vi "Log data.vi"(8 "error in (no error)":errorcluster, 11 "Vessel in":refnum<class "Vessel.lvclass">) -> (0 "error out":errorcluster, 3 "Vessel out":refnum<class "Vessel.lvclass">)   [LabVIEW 2014, in "Vessel.lvclass"]
uses:
  Vessel.lvclass
  <vilib>/imath/engines/lvmath/Plug In/_Char/NIMS_CH_character datatype.ctl
  <vilib>/imath/engines/lvmath2/RunTimeEngine/Managers/WorkSpace/UID Generator.vi
  <vilib>/imath/engines/lvmath/Plug In/_Char/NIMS_CH_String to Character Array.vi
  <vilib>/imath/engines/lvmath2/RunTimeEngine/BuiltInFunctions/length/NIMS_length(GV).vi
  <instcachedir>/0/NIMS_length(GV)_08A3D13377FD4E4B96F5795FBF3698FA.lvgen/NIMS_length(GV)_08A3D13377FD4E4B96F5795FBF3698FA_004.vi
  <vilib>/imath/engines/lvmath2/RunTimeEngine/RunTimeType/NIMS_RunTimeType_From StrictType (excl LVString).vi
  <instcachedir>/0/NIMS_RunTimeType_From StrictType (excl LVString)_15A5391EEA9C4AACB9955AC755B83D29.lvgen/NIMS_RunTimeType_From StrictType (excl LVString)_15A5391EEA9C4AACB9955AC755B83D29_000.vi
  <vilib>/imath/engines/lvmath2/RunTimeEngine/LocalVariableDefStatement/MC_LocalVariableDefStatement_Display.vi
  <vilib>/imath/engines/lvmath2/RunTimeEngine/RangeToken/NIMS_Range_R3 - Integer.vi
  <instcachedir>/0/NIMS_Range_R3 - Integer_66B9031982364693905FDE422E56E490.lvgen/NIMS_Range_R3 - Integer_66B9031982364693905FDE422E56E490_000.vi
  <vilib>/imath/engines/lvmath2/RunTimeEngine/CommandStatement/MC_CommandStatement_break.vi
  <vilib>/imath/engines/lvmath/Plug In/_Char/NIMS_CH_Character 2D to String 1D.vi
  <vilib>/imath/engines/lvmath2/RunTimeEngine/IndexRead/NIMS V(S).vi
  <instcachedir>/0/NIMS V(S)_0488751826AF41519A22953C041130DC.lvgen/NIMS V(S)_0488751826AF41519A22953C041130DC_003.vi
  <vilib>/imath/engines/lvmath2/RunTimeEngine/BuiltInFunctions/strcmp/NIMS_strcmp.vi
  <vilib>/imathl/engines/lvmath/Functions/Error Handling/Create Error.vi
  <vilib>/imath/engines/lvmath2/RunTimeEngine/VariableToken/NIMS_VariableToken_CondDefined.vi
  <instcachedir>/0/NIMS_VariableToken_CondDefined_EE8DD211A89249938CE6537267F5C9B3.lvgen/NIMS_VariableToken_CondDefined_EE8DD211A89249938CE6537267F5C9B3_003.vi
  <vilib>/imath/engines/lvmath2/RunTimeEngine/Managers/SymbolTable/Clear UID.vi
  <vilib>/imath/engines/lvmath2/RunTimeEngine/NodeEndStatement/NIMS_NodeEndStatement_Output.vi
  <instcachedir>/0/NIMS_NodeEndStatement_Output_53EC0D466D134D7ABD903AC30B43404B.lvgen/NIMS_NodeEndStatement_Output_53EC0D466D134D7ABD903AC30B43404B_011.vi
  <vilib>/imath/engines/lvmath2/RunTimeEngine/ErrorHandling/NIMS_Finalize Error.vi
  <vilib>/imath/engines/lvmath2/RunTimeEngine/IndexRead/NIMS V(R2).vi
  <instcachedir>/0/NIMS V(R2)_C76619605A0E4E9F8B2FA9389712AC47.lvgen/NIMS V(R2)_C76619605A0E4E9F8B2FA9389712AC47_002.vi
  <vilib>/imath/engines/lvmath/Plug In/_Char/NIMS_CH_Character RV to String.vi
  <instcachedir>/0/NIMS_NodeEndStatement_Output_53EC0D466D134D7ABD903AC30B43404B.lvgen/NIMS_NodeEndStatement_Output_53EC0D466D134D7ABD903AC30B43404B_009.vi
  Supervisor/Supervisor.lvclass
  <vilib>/imath/engines/lvmath2/RunTimeEngine/Managers/SymbolTable/NIMS_WorkSpace.lvlib
panel:
  out "log line OR":string="21:11:09.2343\t-0.00\t0.00\t30.00\t0.00\t0.00\t-0.00\t0.00\t0.01\t-0.01\t-0.00\t30.00\t0.00\t0.00\t-0.00\t0.00\t0.00\t0.00\t0.00\t30.00\t0.00\t0.00\t0.00\t0.00\t0.00\t132.54\t-43.98\t11.70\t-0.09\t-661 \t252 \t818 \t705 \r\n"
  out "appended path 2":path
  out "appended path":path
  out "log line camera":string="21:11:09.2343\t-0.00\t0.00\t30.00\t0.00\t0.00\t-0.00\t0.00\t0.01\t-0.01\t-0.00\t30.00\t0.00\t0.00\t-0.00\t0.00\t0.00\t0.00\t0.00\t30.00\t0.00\t0.00\t0.00\t0.00\t0.00\t132.54\t-43.98\t11.70\t-0.09\t-661 \t252 \t818 \t705 \r\n"
  out "Start New LogFile":bool
  out "path to log files":string
  out "path 2":path
  out "path":path
  out "log line tau":string="21:11:09.2343\t-0.00\t0.00\t30.00\t0.00\t0.00\t-0.00\t0.00\t0.01\t-0.01\t-0.00\t30.00\t0.00\t0.00\t-0.00\t0.00\t0.00\t0.00\t0.00\t30.00\t0.00\t0.00\t0.00\t0.00\t0.00\t132.54\t-43.98\t11.70\t-0.09\t-661 \t252 \t818 \t705 \r\n"
  out "log line nu":string="21:11:09.2343\t-0.00\t0.00\t30.00\t0.00\t0.00\t-0.00\t0.00\t0.01\t-0.01\t-0.00\t30.00\t0.00\t0.00\t-0.00\t0.00\t0.00\t0.00\t0.00\t30.00\t0.00\t0.00\t0.00\t0.00\t0.00\t132.54\t-43.98\t11.70\t-0.09\t-661 \t252 \t818 \t705 \r\n"
  out "log line eta":string="21:11:09.2343\t-0.00\t0.00\t30.00\t0.00\t0.00\t-0.00\t0.00\t0.01\t-0.01\t-0.00\t30.00\t0.00\t0.00\t-0.00\t0.00\t0.00\t0.00\t0.00\t30.00\t0.00\t0.00\t0.00\t0.00\t0.00\t132.54\t-43.98\t11.70\t-0.09\t-661 \t252 \t818 \t705 \r\n"
  out "log line raw":string="21:11:09.2343\t-0.00\t0.00\t30.00\t0.00\t0.00\t-0.00\t0.00\t0.01\t-0.01\t-0.00\t30.00\t0.00\t0.00\t-0.00\t0.00\t0.00\t0.00\t0.00\t30.00\t0.00\t0.00\t0.00\t0.00\t0.00\t132.54\t-43.98\t11.70\t-0.09\t-661 \t252 \t818 \t705 \r\n"
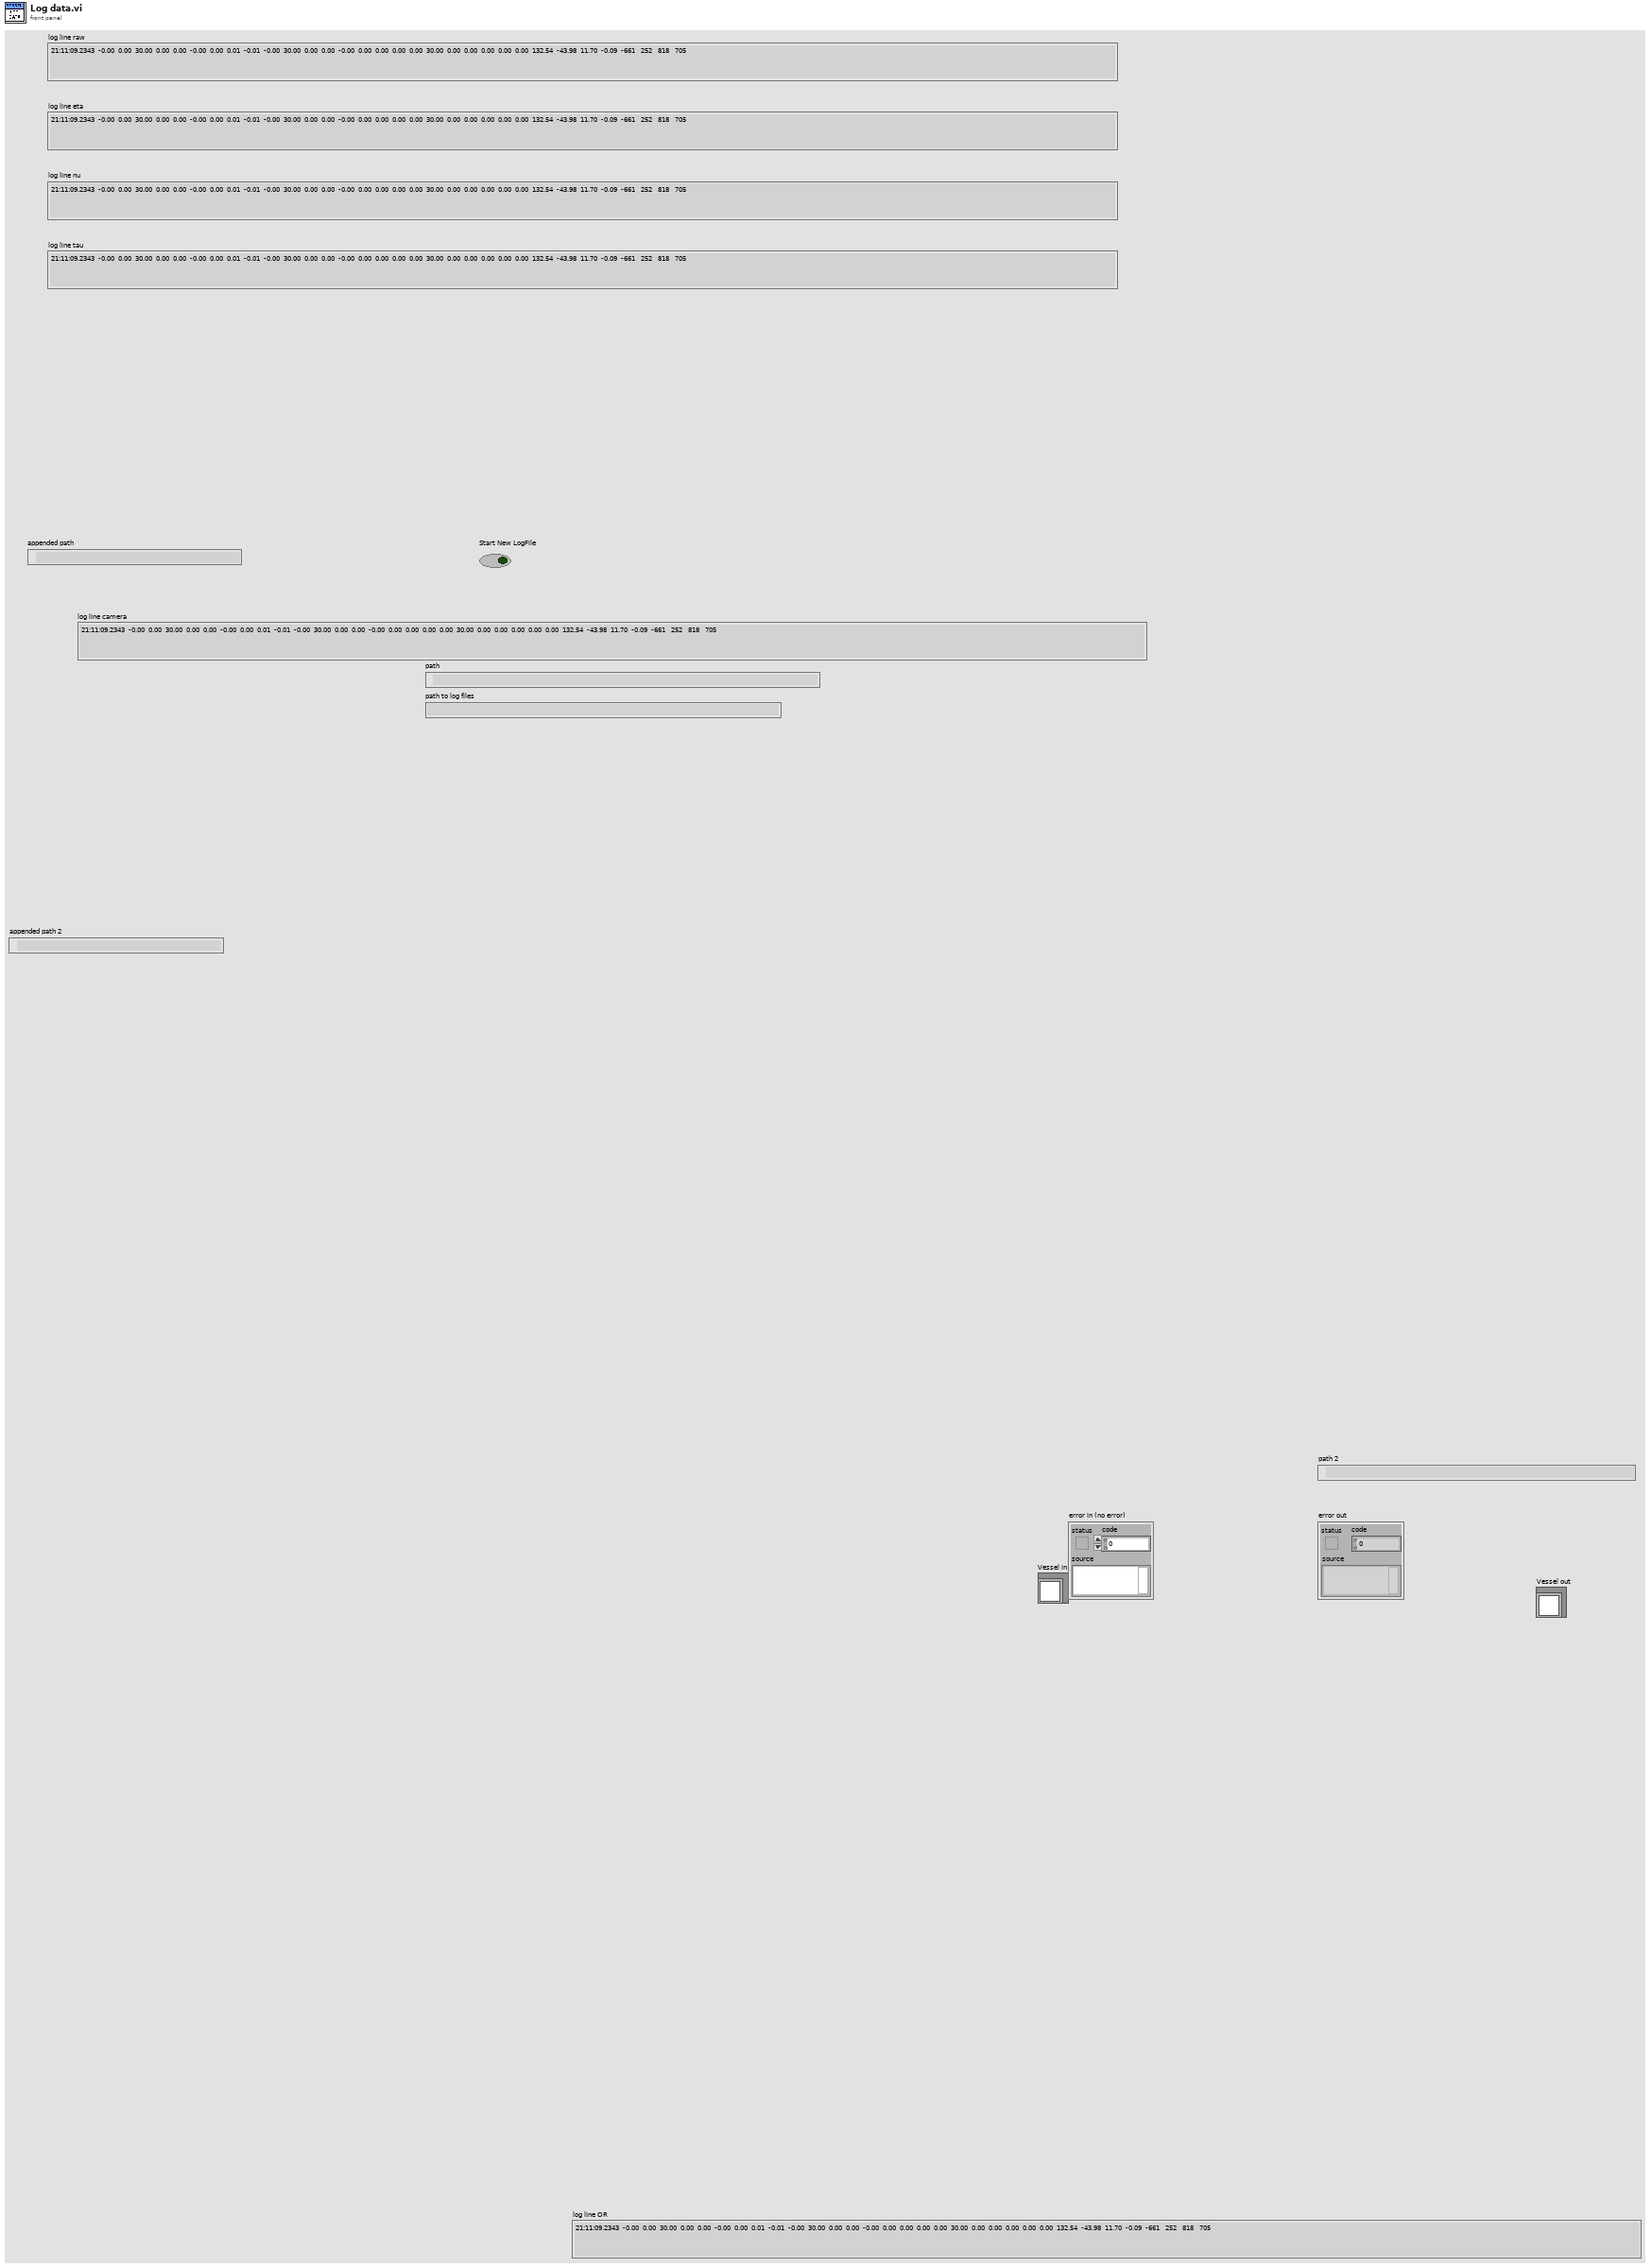
[diagram p1: front panel]
types:
  T1 = enum16{"open", "replace", "create", "open or create", "replace or create", "replace or create with confirmation"}
  T2 = typedef "NIMS_CH_character datatype.ctl" = cluster{"Numeric":u8}
  T3 = cluster{"Measured":cluster{"Eta":dbl[], "Nu":dbl[], "Eta Dot":dbl[], "Nu Dot":dbl[]}, "Estimated":cluster{"Eta":dbl[], "Nu":dbl[], "Eta Dot":dbl[], "Nu Dot":dbl[]}, "Desired":cluster{"Eta":dbl[], "Nu":dbl[], "Eta Dot":dbl[], "Nu Dot":dbl[]}, "Previous Desired":cluster{"Eta":dbl[], "Nu":dbl[], "Eta Dot":dbl[], "Nu Dot":dbl[]}, "tau":dbl[], "Altitude":cluster{"Measured":dbl, "Estimated":dbl, "Desired":dbl, "Previous Desired":dbl, "Approximated":dbl, "grad F":dbl[]}, "rpm":dbl[], "Attitude":cluster{"Theta Measured":dbl[], "Theta Estimated":dbl[], "Omega Measured":dbl[], "Omega Estimated":dbl[], "Gyro Bias":dbl[]}}
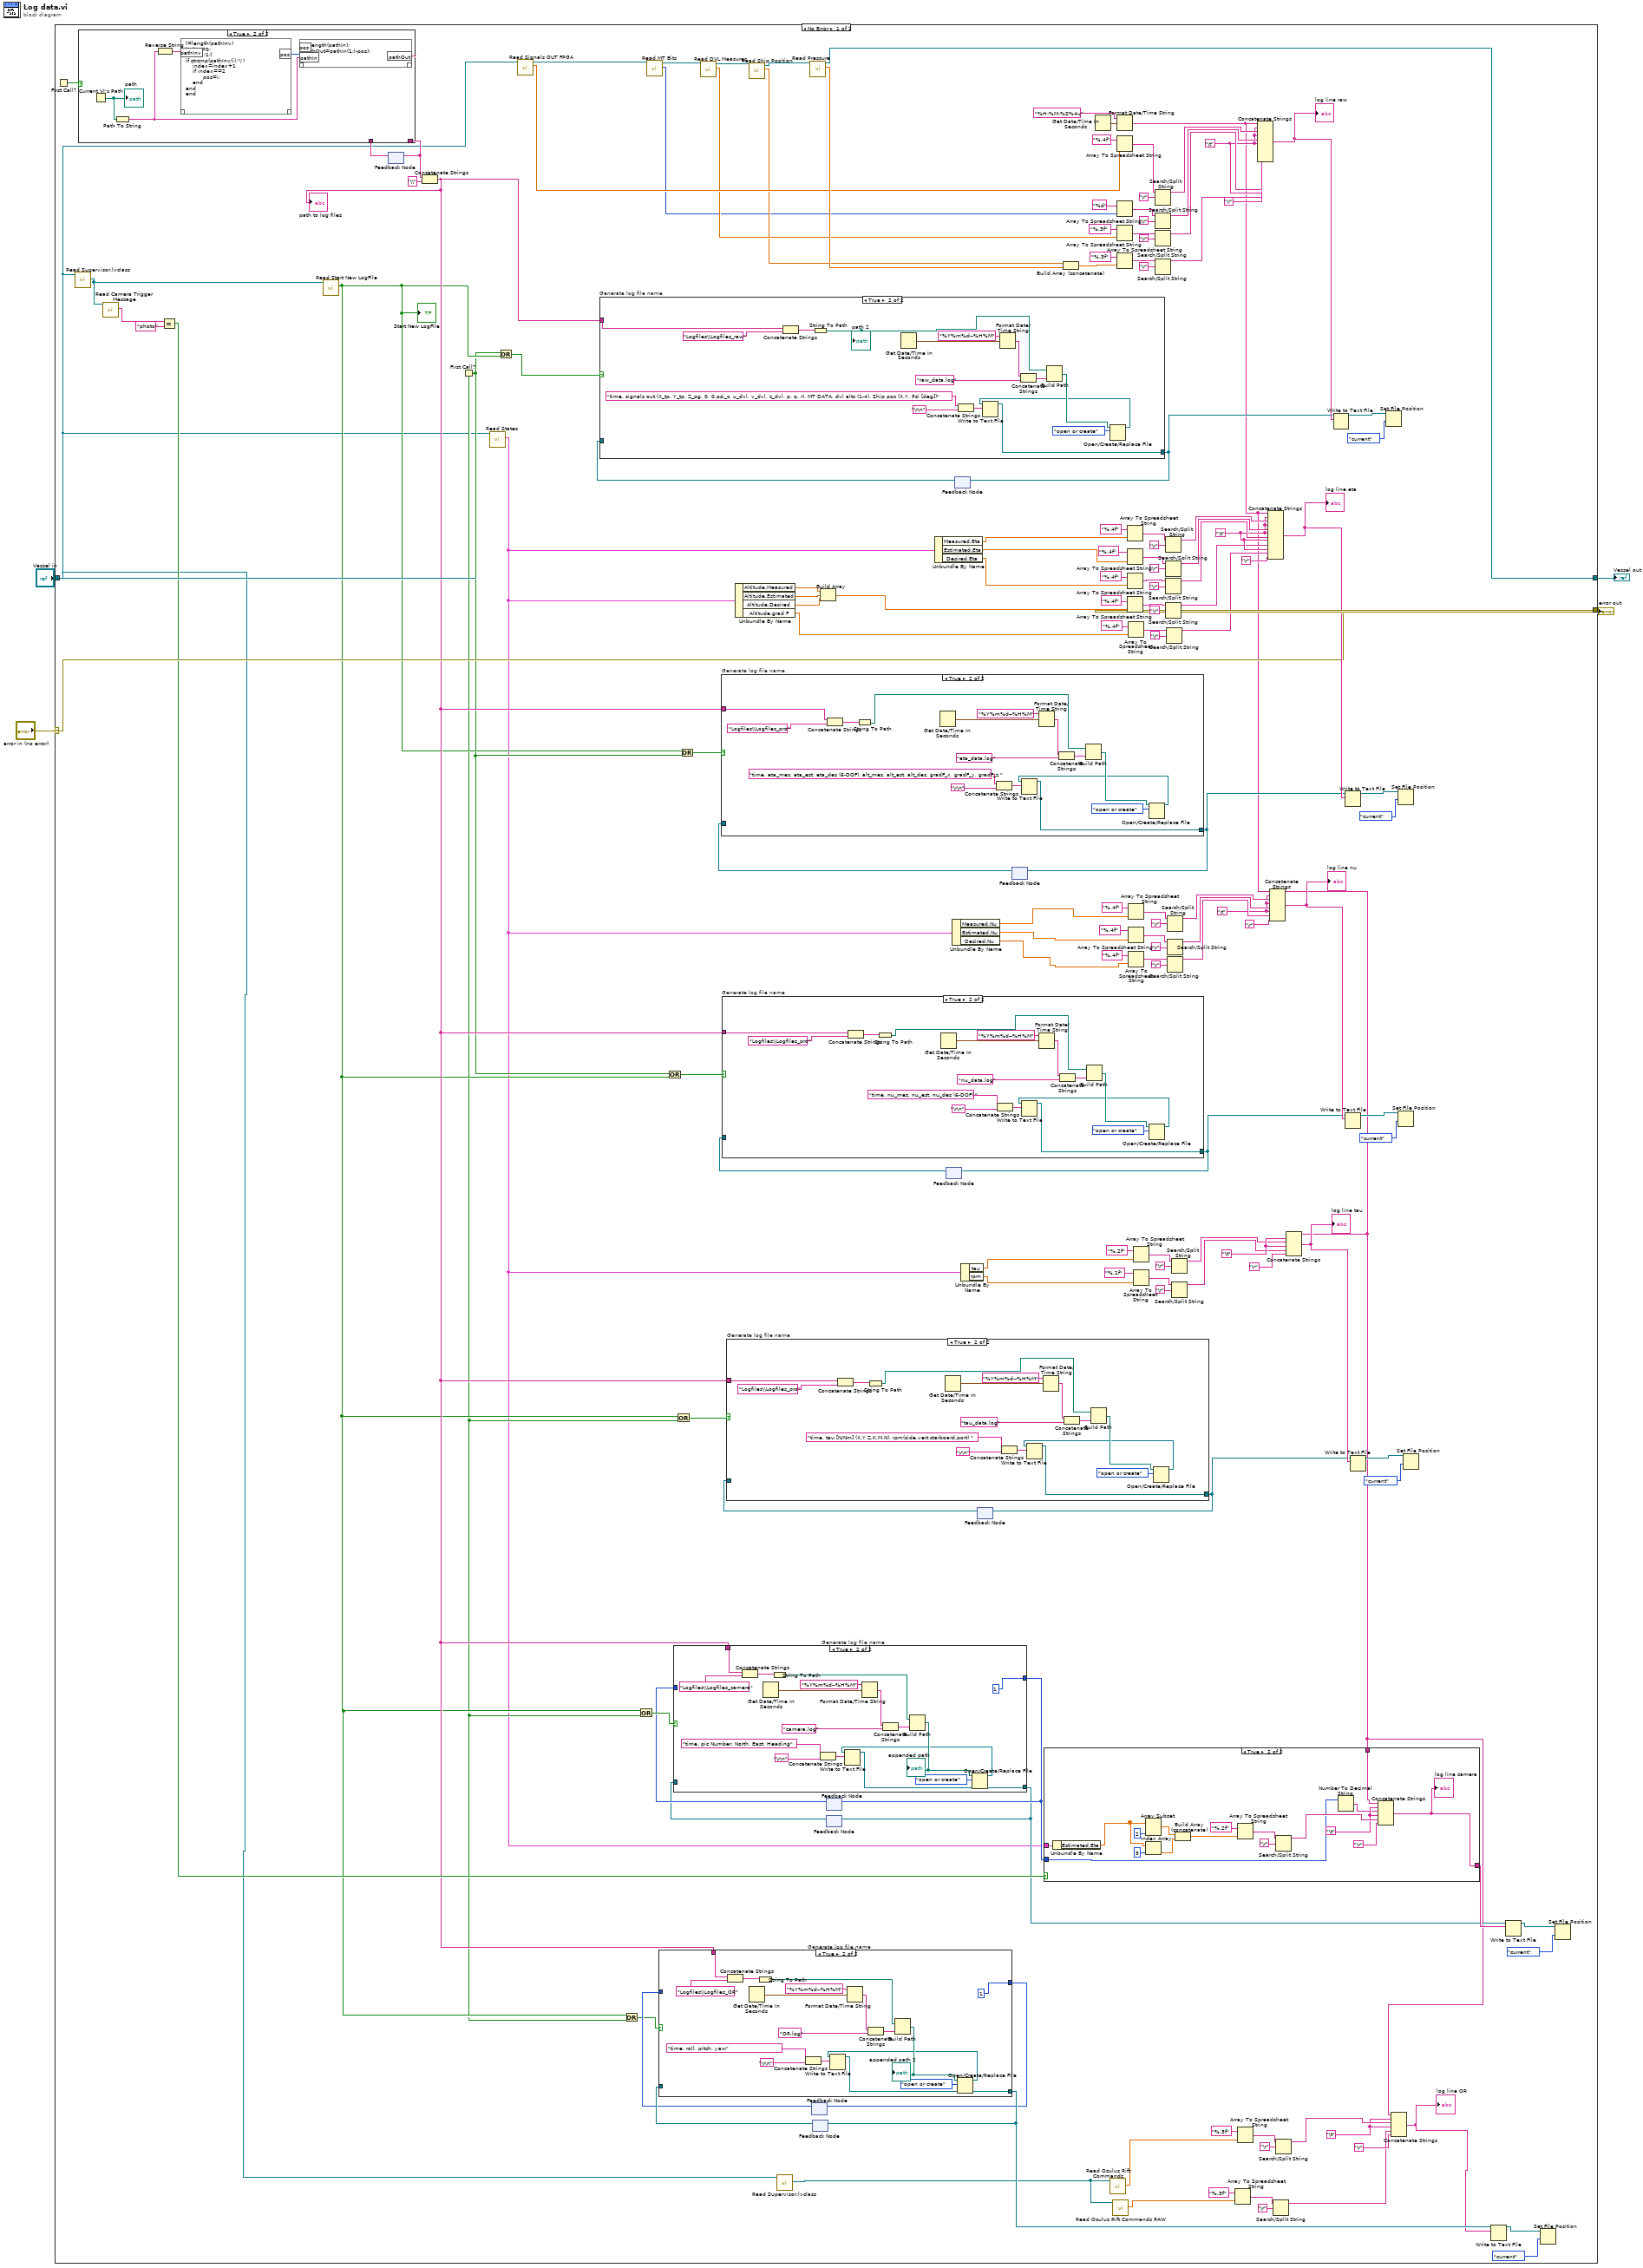
[diagram p0: block diagram]
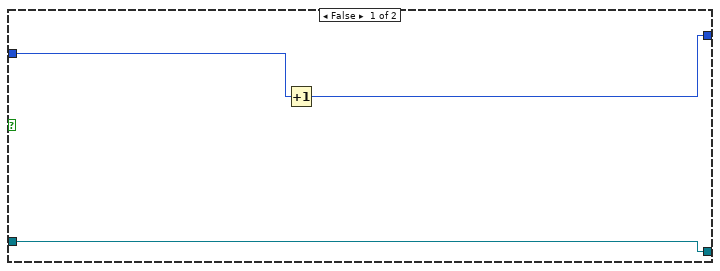
[diagram p2: hidden frame]
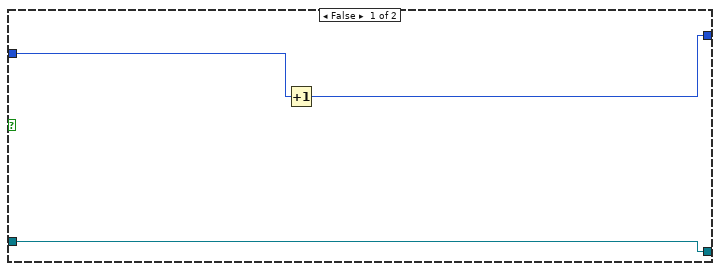
[diagram p3: hidden frame]
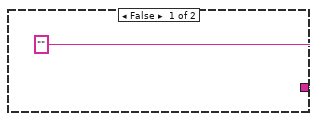
[diagram p4: hidden frame]
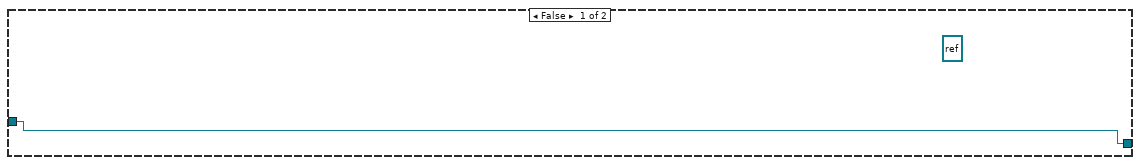
[diagram p9: hidden frame]
diagram:
  n1 = case shown="No Error" "error in (no error)" {
    selector: "error in (no error)" -> [w70 w517]
    tunnel: [w70 w517] -> w1
    tunnel: [w60 w516] -> w3
    tunnel: "Vessel in" -> [w15 w516]
    frame No Error {
      w6 = "\t"
      w87 = "\t"
      w118 = "\t"
      w104 = "\t"
      w74 = "\t"
      n2 = First Call?() -> (First Call?: T/F=w59:bool)
      n3 = call "Read Supervisor.lvclass.vi"("Vessel in"=w15) -> ("Supervisor.lvclass"=w49:refnum<class "Supervisor.lvclass">)  [unwired: 8 in, 2 out]
      n4 = call-dynamic "Read Camera Trigger Message.vi"("Supervisor in"=w49) -> ("Camera Trigger Message"=w48:string)  [unwired: 8 in, 2 out]
      n5 = Equal?(x=w48, y="photo") -> (x = y?=w46:bool)
      n6 = call-dynamic "Read Start New LogFile.vi"("Supervisor in"=w49) -> ("Start New LogFile"=w23:bool)  [unwired: 8 in, 2 out]
      "Start New LogFile" <- w23
      n7 = feedback #1() -> (w58:string)  [unwired: 1 in]
      n8 = case shown="True" w59 {
        tunnel: [w221 w222] -> w57
        tunnel: w58 -> [w221 _]
        frame False {
        }
        frame True {
          n9 = Current VI's Path() -> (path=w226:path)
          "path" <- w226
          n10 = Path To String(path=w226) -> (string=w224:string)
          n11 = Reverse String(1:w224) -> (0:w225:string)
          n12 = mathscript code="l=length(pathInv)\nindex=0;\nfor i=1:1:l\nif strcmp(pathInv(i),'\\')\n    index=index+1\n    if index==2\n          pos=i;\n    end\nend\nend"("pathInv"=w225) -> ("pos"=w223:i32)  [unwired: 1 in, 1 out]
          n13 = mathscript code="l=length(pathIn);\npathOut=pathIn(1:l-pos);"("pathIn"=w224, "pos"=w223) -> ("pathOut"=w222:string)  [unwired: 1 in, 1 out]
        }
      }
      n14 = feedback-in #1(w57) -> ()
      n15 = Concatenate Strings(w57, "\\" ("string")) -> (w24:string)
      "path to log files" <- w24
      n16 = First Call?() -> (First Call?: T/F=w22:bool)
      n17 = call-dynamic "Read States.vi"("Vessel in"=w15) -> ("States"=w17:T3)  [unwired: 8 in, 2 out]
      n18 = Or(x=w22, y=w23) -> (x .or. y?=w55:bool)
      n19 = call-dynamic "Read Signals OUT FPGA.vi"("Vessel in"=w15) -> ("Signals OUT"=w68:dbl[], "Vessel out"=w64:refnum<class "Vessel.lvclass">)  [unwired: 8 in, 1 out]
      n20 = Or(x=w23, y=w22) -> (x .or. y?=w25:bool)
      n21 = Or(x=w23, y=w22) -> (x .or. y?=w45:bool)
      n22 = call-dynamic "Read MT Bits.vi"("Vessel in"=w64) -> ("MT Bits"=w65:u8[], "Vessel out"=w63:refnum<class "Vessel.lvclass">)  [unwired: 8 in, 1 out]
      n23 = Or(x=w22, y=w23) -> (x .or. y?=w54:bool)
      n24 = Or(x=w23, y=w22) -> (x .or. y?=w53:bool)
      n25 = Or(x=w23, y=w22) -> (x .or. y?=w52:bool)
      n26 = call-dynamic "Read DVL Measures.vi"("Vessel in"=w63) -> ("DVL Measures"=w67:dbl[], "Vessel out"=w62:refnum<class "Vessel.lvclass">)  [unwired: 8 in, 1 out]
      n27 = Unbundle By Name(w17) -> ("Altitude.Measured"=w107:dbl, "Altitude.Estimated"=w106:dbl, "Altitude.Desired"=w105:dbl, "Altitude.grad F"=w94:dbl[])
      n28 = call-dynamic "Read Ship Position.vi"("Vessel in"=w62) -> ("Ship Position"=w66:dbl[], "Vessel out"=w61:refnum<class "Vessel.lvclass">)  [unwired: 8 in, 1 out]
      n29 = call "Read Supervisor.lvclass.vi"("Vessel in"=w15) -> ("Supervisor.lvclass"=w11:refnum<class "Supervisor.lvclass">)  [unwired: 8 in, 2 out]
      n30 = call-dynamic "Read Pressure.vi"("Vessel in"=w61) -> ("Pressure"=w69:dbl, "Vessel out"=w60:refnum<class "Vessel.lvclass">)  [unwired: 8 in, 1 out]
      n31 = feedback #2() -> (w26:i32)  [unwired: 1 in]
      n32 = feedback #3() -> (w31:refnum<file>)  [unwired: 1 in]
      n33 = case "Generate log file name" shown="True" w25 {
        tunnel: [w163 w172] -> w30
        tunnel: w24 -> [_ w167]
        tunnel: [w164 1] -> w27
        tunnel: w26 -> [w165 _]
        tunnel: w31 -> [w163 _]
        frame False {
          n34 = Increment(x=w165) -> (x+1=w164:i32)
        }
        frame True {
          n35 = Concatenate Strings(w167, "Logfiles\\Logfiles_OR" ("string")) -> (w169:string)
          n36 = Get Date/Time In Seconds() -> (seconds since 1Jan1904=w179:timestamp)
          n37 = String To Path(string=w169) -> (path=w168:path)
          n38 = Concatenate Strings("time, roll, pitch, yaw" ("string"), "\r\n") -> (w174:string)
          n39 = Format Date/Time String(time format string (%c)="%Y%m%d--%H%M", seconds (now)=w179) -> (date/time string=w177:string)  [unwired: 1 in]
          n40 = Concatenate Strings(w177, "OR.log" ("string")) -> (w181:string)
          n41 = Build Path(base path=w168, name or relative path=w181) -> (appended path=w180:path)
          "appended path 2" <- w180
          n42 = Open/Create/Replace File(file path (use dialog)=w180, operation (0:open)=T1."open or create") -> (refnum out=w173:refnum<file>)  [unwired: 4 in, 2 out]
          n43 = Write to Text File(file (use dialog)=w173, text=w174) -> (refnum out=w172:refnum<file>)  [unwired: 2 in, 2 out]
        }
      }
      n44 = feedback-in #2(w27) -> ()
      n45 = feedback-in #3(w30) -> ()
      n46 = Build Array(w107, w106, w105) -> (w100:dbl[])
      n47 = feedback #4() -> (w44:i32)  [unwired: 1 in]
      n48 = feedback #5() -> (w38:refnum<file>)  [unwired: 1 in]
      n49 = case "Generate log file name" shown="True" w45 {
        tunnel: [w183 w192] -> w39
        tunnel: w24 -> [_ w187]
        tunnel: [w184 1] -> w43
        tunnel: w44 -> [w185 _]
        tunnel: w38 -> [w183 _]
        frame False {
          n50 = Increment(x=w185) -> (x+1=w184:i32)
        }
        frame True {
          n51 = Concatenate Strings(w187, "Logfiles\\Logfiles_camera" ("string")) -> (w189:string)
          n52 = Get Date/Time In Seconds() -> (seconds since 1Jan1904=w199:timestamp)
          n53 = String To Path(string=w189) -> (path=w188:path)
          n54 = Concatenate Strings("time, pic Number, North, East, Heading" ("string"), "\r\n") -> (w194:string)
          n55 = Format Date/Time String(time format string (%c)="%Y%m%d--%H%M", seconds (now)=w199) -> (date/time string=w197:string)  [unwired: 1 in]
          n56 = Concatenate Strings(w197, "camera.log" ("string")) -> (w201:string)
          n57 = Build Path(base path=w188, name or relative path=w201) -> (appended path=w200:path)
          "appended path" <- w200
          n58 = Open/Create/Replace File(file path (use dialog)=w200, operation (0:open)=T1."open or create") -> (refnum out=w193:refnum<file>)  [unwired: 4 in, 2 out]
          n59 = Write to Text File(file (use dialog)=w193, text=w194) -> (refnum out=w192:refnum<file>)  [unwired: 2 in, 2 out]
        }
      }
      n60 = feedback-in #4(w43) -> ()
      n61 = feedback-in #5(w39) -> ()
      n62 = Unbundle By Name(w17) -> ("Measured.Eta"=w113:dbl[], "Estimated.Eta"=w112:dbl[], "Desired.Eta"=w111:dbl[])
      n63 = feedback #6() -> (w36:refnum<file>)  [unwired: 1 in]
      n64 = case "Generate log file name" shown="True" w54 {
        tunnel: [w465 w471] -> w35
        tunnel: w24 -> [_ w467]
        tunnel: w36 -> [w465 _]
        frame False {
        }
        frame True {
          n65 = Concatenate Strings(w467, "Logfiles\\Logfiles_pro" ("string")) -> (w468:string)
          n66 = String To Path(string=w468) -> (path=w466:path)
          n67 = Get Date/Time In Seconds() -> (seconds since 1Jan1904=w478:timestamp)
          n68 = Concatenate Strings("time, nu_mes, nu_est, nu_des (6-DOF) " ("string"), "\r\n") -> (w473:string)
          n69 = Format Date/Time String(time format string (%c)="%Y%m%d--%H%M", seconds (now)=w478) -> (date/time string=w476:string)  [unwired: 1 in]
          n70 = Concatenate Strings(w476, "nu_data.log" ("string")) -> (w480:string)
          n71 = Build Path(base path=w466, name or relative path=w480) -> (appended path=w479:path)
          n72 = Open/Create/Replace File(file path (use dialog)=w479, operation (0:open)=T1."open or create") -> (refnum out=w472:refnum<file>)  [unwired: 4 in, 2 out]
          n73 = Write to Text File(file (use dialog)=w472, text=w473) -> (refnum out=w471:refnum<file>)  [unwired: 2 in, 2 out]
        }
      }
      n74 = feedback-in #6(w35) -> ()
      n75 = Unbundle By Name(w17) -> ("Measured.Nu"=w110:dbl[], "Estimated.Nu"=w109:dbl[], "Desired.Nu"=w108:dbl[])
      n76 = feedback #7() -> (w51:refnum<file>)  [unwired: 1 in]
      n77 = case "Generate log file name" shown="True" w55 {
        tunnel: [w499 w504] -> w50
        tunnel: w24 -> [_ w502]
        tunnel: w51 -> [w499 _]
        frame False {
          (unwired) refnum<file> refnum ("refnum out")
        }
        frame True {
          n78 = Concatenate Strings(w502, "Logfiles\\Logfiles_raw" ("string")) -> (w501:string)
          n79 = String To Path(string=w501) -> (path=w500:path)
          "path 2" <- w500
          n80 = Get Date/Time In Seconds() -> (seconds since 1Jan1904=w512:timestamp)
          n81 = Concatenate Strings("time, signals out (X_tp, Y_tp, Z_pg, 0, 0,psi_c, u_dvl, v_dvl, z_dvl, p, q, r), MT DATA, dvl alts (1-4), Ship pos (X,Y, Psi [deg])" ("string"), "\r\n") -> (w506:string)
          n82 = Format Date/Time String(time format string (%c)="%Y%m%d--%H%M", seconds (now)=w512) -> (date/time string=w510:string)  [unwired: 1 in]
          n83 = Concatenate Strings(w510, "raw_data.log" ("string")) -> (w514:string)
          n84 = Build Path(base path=w500, name or relative path=w514) -> (appended path=w513:path)
          n85 = Open/Create/Replace File(file path (use dialog)=w513, operation (0:open)=T1."open or create") -> (refnum out=w505:refnum<file>)  [unwired: 4 in, 2 out]
          n86 = Write to Text File(file (use dialog)=w505, text=w506) -> (refnum out=w504:refnum<file>)  [unwired: 2 in, 2 out]
        }
      }
      n87 = feedback-in #7(w50) -> ()
      n88 = Unbundle By Name(w17) -> ("tau"=w91:dbl[], "rpm"=w92:dbl[])
      n89 = feedback #8() -> (w37:refnum<file>)  [unwired: 1 in]
      n90 = case "Generate log file name" shown="True" w53 {
        tunnel: [w448 w454] -> w32
        tunnel: w24 -> [_ w450]
        tunnel: w37 -> [w448 _]
        frame False {
        }
        frame True {
          n91 = Concatenate Strings(w450, "Logfiles\\Logfiles_pro" ("string")) -> (w451:string)
          n92 = String To Path(string=w451) -> (path=w449:path)
          n93 = Get Date/Time In Seconds() -> (seconds since 1Jan1904=w461:timestamp)
          n94 = Concatenate Strings("time, tau [N/Nm] (X,Y,Z,K,M,N), rpm(side,vert,starboard,port) " ("string"), "\r\n") -> (w456:string)
          n95 = Format Date/Time String(time format string (%c)="%Y%m%d--%H%M", seconds (now)=w461) -> (date/time string=w459:string)  [unwired: 1 in]
          n96 = Concatenate Strings(w459, "tau_data.log" ("string")) -> (w463:string)
          n97 = Build Path(base path=w449, name or relative path=w463) -> (appended path=w462:path)
          n98 = Open/Create/Replace File(file path (use dialog)=w462, operation (0:open)=T1."open or create") -> (refnum out=w455:refnum<file>)  [unwired: 4 in, 2 out]
          n99 = Write to Text File(file (use dialog)=w455, text=w456) -> (refnum out=w454:refnum<file>)  [unwired: 2 in, 2 out]
        }
      }
      n100 = feedback-in #8(w32) -> ()
      n101 = feedback #9() -> (w34:refnum<file>)  [unwired: 1 in]
      n102 = case "Generate log file name" shown="True" w52 {
        tunnel: [w482 w487] -> w33
        tunnel: w24 -> [_ w484]
        tunnel: w34 -> [w482 _]
        frame False {
        }
        frame True {
          n103 = Concatenate Strings(w484, "Logfiles\\Logfiles_pro" ("string")) -> (w485:string)
          n104 = String To Path(string=w485) -> (path=w483:path)
          n105 = Get Date/Time In Seconds() -> (seconds since 1Jan1904=w495:timestamp)
          n106 = Concatenate Strings("time, eta_mes, eta_est, eta_des (6-DOF), alt_mes, alt_est, alt_des, gradF_x, gradF_y, gradF_z " ("string"), "\r\n") -> (w489:string)
          n107 = Format Date/Time String(time format string (%c)="%Y%m%d--%H%M", seconds (now)=w495) -> (date/time string=w493:string)  [unwired: 1 in]
          n108 = Concatenate Strings(w493, "eta_data.log" ("string")) -> (w497:string)
          n109 = Build Path(base path=w483, name or relative path=w497) -> (appended path=w496:path)
          n110 = Open/Create/Replace File(file path (use dialog)=w496, operation (0:open)=T1."open or create") -> (refnum out=w488:refnum<file>)  [unwired: 4 in, 2 out]
          n111 = Write to Text File(file (use dialog)=w488, text=w489) -> (refnum out=w487:refnum<file>)  [unwired: 2 in, 2 out]
        }
      }
      n112 = feedback-in #9(w33) -> ()
      n113 = Build Array (concatenate)(w66, w69) -> (w71:dbl[])
      n114 = Get Date/Time In Seconds() -> (seconds since 1Jan1904=w152:timestamp)
      n115 = call-dynamic "Read Oculus Rift Commands.vi"("Supervisor in"=w11) -> ("Oculus Rift Commands"=w14:dbl[])  [unwired: 8 in, 2 out]
      n116 = call-dynamic "Read Oculus Rift Commands RAW.vi"("Supervisor in"=w11) -> ("Oculus Rift Commands RAW"=w7:dbl[])  [unwired: 8 in, 2 out]
      n117 = Format Date/Time String(time format string (%c)="%H:%M:%S%4u", seconds (now)=w152) -> (date/time string=w12:string)  [unwired: 1 in]
      n118 = case shown="True" w46 {
        tunnel: w17 -> [_ w216]
        tunnel: w12 -> [_ w208]
        tunnel: w43 -> [_ w205]
        tunnel: ["" w204] -> w40
        frame False {
        }
        frame True {
          w207 = "\t"
          n119 = Unbundle By Name(w216) -> ("Estimated.Eta"=w213:dbl[])
          n120 = Array Subset(array=w213, length=2) -> (w212:dbl[])  [unwired: 1 in]
          n121 = Index Array(array=w213, index=5) -> (element=w211:dbl)
          n122 = Build Array (concatenate)(w212, w211) -> (w210:dbl[])
          n123 = Array To Spreadsheet String(array=w210, 3:"%.2f" ("format string")) -> (spreadsheet string=w217:string)  [unwired: 1 in]
          n124 = Search/Split String(string=w217, search string/char (-)="\r") -> (substring before match=w218:string)  [unwired: 1 in, 2 out]
          n125 = Number To Decimal String(number=w205) -> (decimal integer string=w206:string)  [unwired: 1 in]
          n126 = Concatenate Strings(w208, w207, w206, w207, w218, "\r") -> (w204:string)
          "log line camera" <- w204
        }
      }
      n127 = Array To Spreadsheet String(array=w68, 3:"%.4f" ("format string")) -> (spreadsheet string=w147:string)  [unwired: 1 in]
      n128 = Array To Spreadsheet String(array=w65, 3:"%d" ("format string")) -> (spreadsheet string=w146:string)  [unwired: 1 in]
      n129 = Array To Spreadsheet String(array=w67, 3:"%.3f" ("format string")) -> (spreadsheet string=w158:string)  [unwired: 1 in]
      n130 = Array To Spreadsheet String(array=w71, 3:"%.3f" ("format string")) -> (spreadsheet string=w77:string)  [unwired: 1 in]
      n131 = Array To Spreadsheet String(array=w113, 3:"%.4f" ("format string")) -> (spreadsheet string=w144:string)  [unwired: 1 in]
      n132 = Array To Spreadsheet String(array=w112, 3:"%.4f" ("format string")) -> (spreadsheet string=w145:string)  [unwired: 1 in]
      n133 = Array To Spreadsheet String(array=w111, 3:"%.4f" ("format string")) -> (spreadsheet string=w102:string)  [unwired: 1 in]
      n134 = Array To Spreadsheet String(array=w100, 3:"%.4f" ("format string")) -> (spreadsheet string=w95:string)  [unwired: 1 in]
      n135 = Array To Spreadsheet String(array=w94, 3:"%.4f" ("format string")) -> (spreadsheet string=w97:string)  [unwired: 1 in]
      n136 = Array To Spreadsheet String(array=w110, 3:"%.4f" ("format string")) -> (spreadsheet string=w115:string)  [unwired: 1 in]
      n137 = Array To Spreadsheet String(array=w109, 3:"%.4f" ("format string")) -> (spreadsheet string=w114:string)  [unwired: 1 in]
      n138 = Array To Spreadsheet String(array=w108, 3:"%.4f" ("format string")) -> (spreadsheet string=w125:string)  [unwired: 1 in]
      n139 = Array To Spreadsheet String(array=w91, 3:"%.2f" ("format string")) -> (spreadsheet string=w89:string)  [unwired: 1 in]
      n140 = Array To Spreadsheet String(array=w92, 3:"%.1f" ("format string")) -> (spreadsheet string=w90:string)  [unwired: 1 in]
      n141 = Search/Split String(string=w147, search string/char (-)="\r") -> (substring before match=w157:string)  [unwired: 1 in, 2 out]
      n142 = Search/Split String(string=w146, search string/char (-)="\r") -> (substring before match=w156:string)  [unwired: 1 in, 2 out]
      n143 = Search/Split String(string=w158, search string/char (-)="\r") -> (substring before match=w155:string)  [unwired: 1 in, 2 out]
      n144 = Search/Split String(string=w77, search string/char (-)="\r") -> (substring before match=w73:string)  [unwired: 1 in, 2 out]
      n145 = Search/Split String(string=w144, search string/char (-)="\r") -> (substring before match=w136:string)  [unwired: 1 in, 2 out]
      n146 = Search/Split String(string=w145, search string/char (-)="\r") -> (substring before match=w137:string)  [unwired: 1 in, 2 out]
      n147 = Search/Split String(string=w102, search string/char (-)="\r") -> (substring before match=w138:string)  [unwired: 1 in, 2 out]
      n148 = Search/Split String(string=w95, search string/char (-)="\r") -> (substring before match=w99:string)  [unwired: 1 in, 2 out]
      n149 = Search/Split String(string=w97, search string/char (-)="\r") -> (substring before match=w93:string)  [unwired: 1 in, 2 out]
      n150 = Search/Split String(string=w115, search string/char (-)="\r") -> (substring before match=w124:string)  [unwired: 1 in, 2 out]
      n151 = Search/Split String(string=w114, search string/char (-)="\r") -> (substring before match=w123:string)  [unwired: 1 in, 2 out]
      n152 = Search/Split String(string=w125, search string/char (-)="\r") -> (substring before match=w122:string)  [unwired: 1 in, 2 out]
      n153 = Search/Split String(string=w89, search string/char (-)="\r") -> (substring before match=w83:string)  [unwired: 1 in, 2 out]
      n154 = Search/Split String(string=w90, search string/char (-)="\r") -> (substring before match=w84:string)  [unwired: 1 in, 2 out]
      n155 = Array To Spreadsheet String(array=w7, 3:"%.3f" ("format string")) -> (spreadsheet string=w8:string)  [unwired: 1 in]
      n156 = Array To Spreadsheet String(array=w14, 3:"%.3f" ("format string")) -> (spreadsheet string=w21:string)  [unwired: 1 in]
      n157 = Concatenate Strings(w12, w74, w157, w74, w156, w74, w155, w74, w73, "\r") -> (w149:string)
      "log line raw" <- w149
      n158 = Concatenate Strings(w12, w104, w136, w104, w137, w104, w138, w104, w99, w104, w93, "\r") -> (w143:string)
      "log line eta" <- w143
      n159 = Concatenate Strings(w12, w118, w124, w118, w123, w118, w122, "\r") -> (w116:string)
      "log line nu" <- w116
      n160 = Search/Split String(string=w8, search string/char (-)="\r") -> (substring before match=w5:string)  [unwired: 1 in, 2 out]
      n161 = Search/Split String(string=w21, search string/char (-)="\r") -> (substring before match=w20:string)  [unwired: 1 in, 2 out]
      n162 = Concatenate Strings(w12, w87, w83, w87, w84, "\r") -> (w88:string)
      "log line tau" <- w88
      n163 = Write to Text File(file (use dialog)=w50, text=w149) -> (refnum out=w151:refnum<file>)  [unwired: 2 in, 2 out]
      n164 = Write to Text File(file (use dialog)=w33, text=w143) -> (refnum out=w140:refnum<file>)  [unwired: 2 in, 2 out]
      n165 = Write to Text File(file (use dialog)=w35, text=w116) -> (refnum out=w120:refnum<file>)  [unwired: 2 in, 2 out]
      n166 = Write to Text File(file (use dialog)=w32, text=w88) -> (refnum out=w85:refnum<file>)  [unwired: 2 in, 2 out]
      n167 = Set File Position(refnum=w151, from (0:start)=enum16{"start", "end", "current"}."current") -> ()  [unwired: 2 in, 2 out]
      n168 = Concatenate Strings(w12, w6, w20, w6, w5, "\r") -> (w16:string)
      "log line OR" <- w16
      n169 = Set File Position(refnum=w140, from (0:start)=enum16{"start", "end", "current"}."current") -> ()  [unwired: 2 in, 2 out]
      n170 = Set File Position(refnum=w120, from (0:start)=enum16{"start", "end", "current"}."current") -> ()  [unwired: 2 in, 2 out]
      n171 = Set File Position(refnum=w85, from (0:start)=enum16{"start", "end", "current"}."current") -> ()  [unwired: 2 in, 2 out]
      n172 = Write to Text File(file (use dialog)=w30, text=w16) -> (refnum out=w28:refnum<file>)  [unwired: 2 in, 2 out]
      n173 = Write to Text File(file (use dialog)=w39, text=w40) -> (refnum out=w42:refnum<file>)  [unwired: 2 in, 2 out]
      n174 = Set File Position(refnum=w28, from (0:start)=enum16{"start", "end", "current"}."current") -> ()  [unwired: 2 in, 2 out]
      n175 = Set File Position(refnum=w42, from (0:start)=enum16{"start", "end", "current"}."current") -> ()  [unwired: 2 in, 2 out]
    }
    frame Error {
    }
  }
  "Vessel out" <- w3
  "error out" <- w1
